vi "cs_saveStimList.vi"(4 "error in (no error)":errorcluster, 6 "Path In":path, 7 "Stimulus List":dbl[][](array[numeric])) -> (0 "error out":errorcluster, 2 "Path":path)   [LabVIEW 2013]
uses:
  <vilib>/Utility/xml.llb/Write to XML File(array).vi
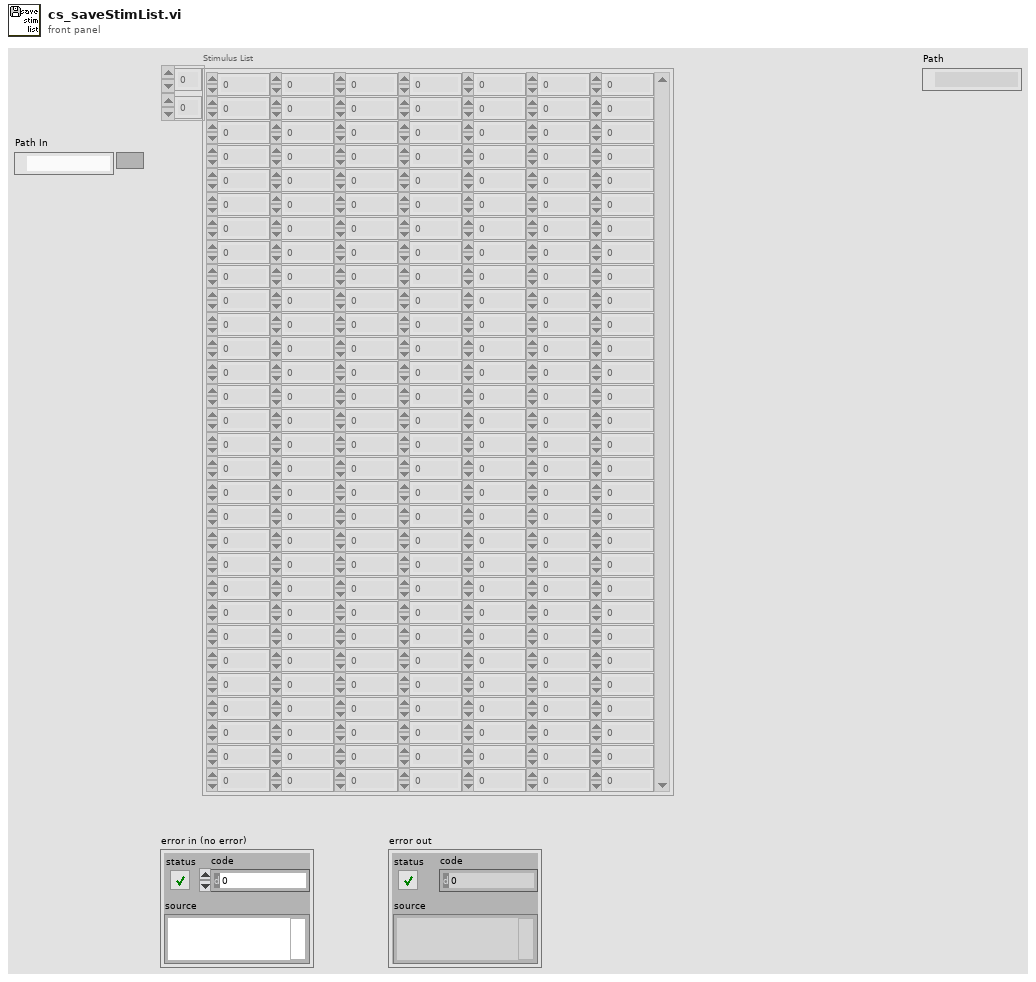
[diagram p1: front panel]
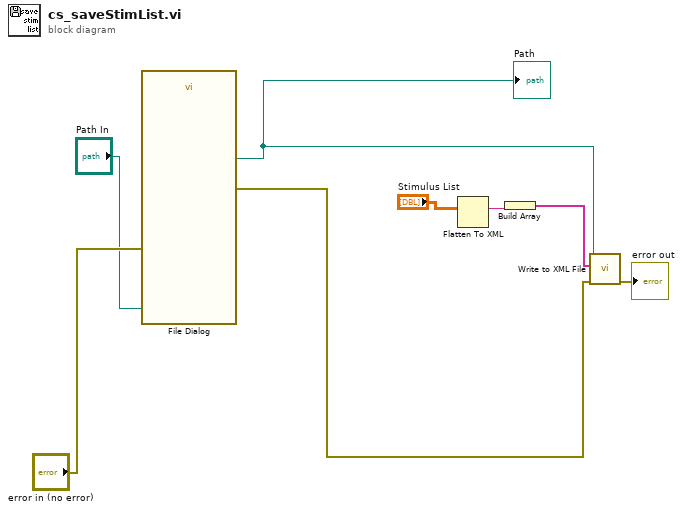
[diagram p0: block diagram]
diagram:
  n1 = call "File Dialog"("start path"="Path In", "error in"="error in (no error)") -> ("selected path"=w7:path, "error out"=w5:errorcluster)  [unwired: 10 in, 2 out]
  "Path" <- w7
  n2 = Flatten To XML(anything="Stimulus List") -> (xml string=w3:string)
  n3 = Build Array(w3) -> (w2:string[])
  n4 = call-poly <vilib>:"Write to XML File.vi"("error in (no error)"=w5, "XML Input"=w2, "XML File Path"=w7) -> ("error out"=→"error out":errorcluster)  [unwired: 6 in, 2 out]
